vi "init_Kloehn.vi"() -> ()   [LabVIEW 2010]
panel:
  out "error out":errorcluster
  in  "init?":bool=TRUE
  in  "VISA resource name":refnum<visa-resource-name>="COM10"
  in  "error in":errorcluster
  in  "Port Configuration":T1={"baud rate (9600)"=9600, "data bits (8)"=8, "parity (0:none)"=enum."None", "stop bits (10: 1 bit)"=10, "flow control (0:none)"=0, "timeout (10sec)"=10000, "termination char\n(0xA = '\\n' = LF) "=10, "Enable Termination\nChar (T)"=TRUE} {"termination char\n(0xA = '\\n' = LF)" format="%.0x"; "flow control (0:none)" items=["None", "XON/XOFF", "RTS/CTS", "XON/XOFF & RTS/CTS", "DTR/DSR", "XON/XOFF & DTR/DSR"]; "stop bits (10: 1 bit)" items=["1.0"=10, "1.5"=15, "2.0"=20]; "data bits (8)" min=5 max=8 step=1}
  # "]"
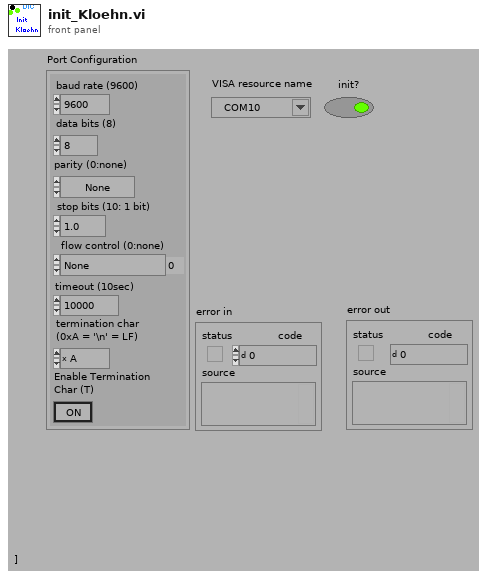
[diagram p1: front panel]
types:
  T1 = cluster{"baud rate (9600)":u32, "data bits (8)":u16, "parity (0:none)":enum16{"None", "Odd", "Even", "Mark", "Space"}, "stop bits (10: 1 bit)":u16, "flow control (0:none)":u16, "timeout (10sec)":u32, "termination char\n(0xA = '\\n' = LF) ":u8, "Enable Termination\nChar (T)":bool}
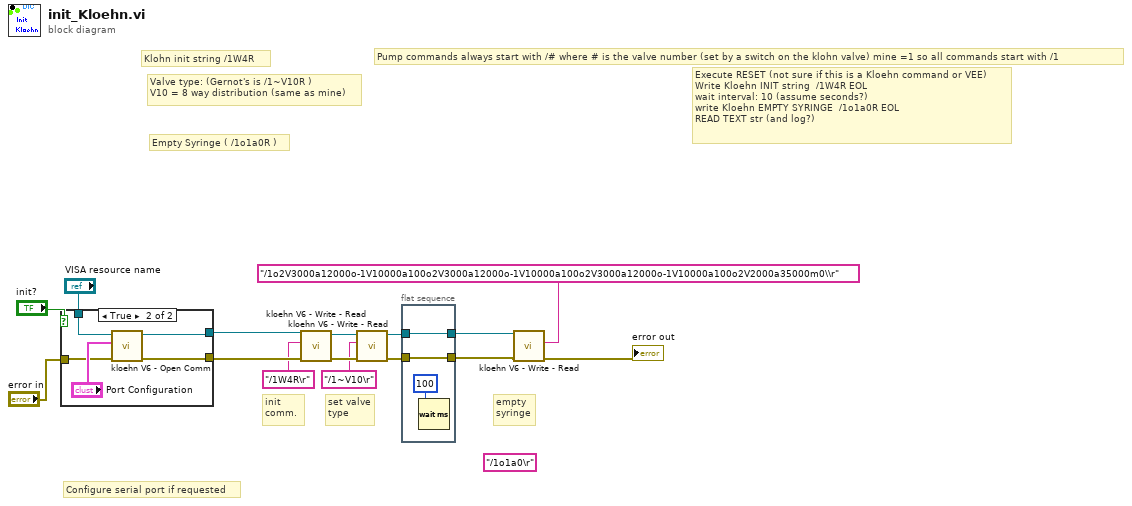
[diagram p0: block diagram]
diagram:
  (unwired) "/1o1a0\r" ("Send String")
  # "empty\nsyringe"
  # "set valve\ntype"
  # "init\ncomm."
  # "Pump commands always start with /# where # is the valve number (set by a switch on the klohn valve) mine =1 so all commands start with /1"
  # "Configure serial port if requested"
  # "Execute RESET (not sure if this is a Kloehn command or VEE)\nWrite Kloehn INIT string  /1W4R EOL\nwait interval: 10 (assume seconds?)\nwrite Kloehn EMPTY SYRINGE  /1o1a0R EOL\nREAD TEXT str (and log?)"
  # "Empty Syringe ( /1o1a0R )"
  # "Valve type: (Gernot's is /1~V10R )\nV10 = 8 way distribution (same as mine)"
  # "Klohn init string /1W4R"
  n1 = case shown="True" "init?" {
    tunnel: [w16 w19] -> w12
    tunnel: [w17 w18] -> w11
    tunnel: "error in" -> [w17 w21]
    tunnel: "VISA resource name" -> [w16 w20]
    frame False {
    }
    frame True {
      n2 = call "kloehn V6 - Open Comm .vi"("error in"=w21, "Serial Parameters"="Port Configuration", "VISA Ref"=w20) -> ("error out"=w18:errorcluster, "VISA Ref DUP"=w19:refnum<visa-resource-name>)  [unwired: 7 in]
    }
  }
  n3 = call "kloehn V6 - Write - Read.vi"("error in"=w11, "Send String"="/1W4R\r", "VISA Ref"=w12) -> ("error out"=w9:errorcluster, "VISA Ref DUP"=w8:refnum<visa-resource-name>)  [unwired: 4 in, 3 out]
  n4 = call "kloehn V6 - Write - Read.vi"("error in"=w9, "Send String"="/1~V10\r", "VISA Ref"=w8) -> ("error out"=w6:errorcluster, "VISA Ref DUP"=w4:refnum<visa-resource-name>)  [unwired: 4 in, 3 out]
  n5 = flat-sequence {
    tunnel: w4 -> [w25]
    tunnel: [w25] -> w3
    tunnel: w6 -> [w23]
    tunnel: [w23] -> w5
    frame #0 {
      n6 = Wait (ms)(milliseconds to wait=100) -> ()  [unwired: 1 out]
    }
  }
  n7 = call "kloehn V6 - Write - Read.vi"("error in"=w5, "Send String"="/1o2V3000a12000o-1V10000a100o2V3000a12000o-1V10000a100o2V3000a12000o-1V10000a100o2V2000a35000m0\\r", "VISA Ref"=w3) -> ("error out"=→"error out":errorcluster)  [unwired: 4 in, 4 out]
